vi "Clear Plots Without Assigned Variables.vi"(8 "error in":errorcluster, 10 "Plot Channel Configurations":T3[](array[typedef]), 11 "Plot Data In":T1[](array[typedef])) -> (0 "error out":errorcluster, 3 "Plot Data Out":T1[](array[typedef]))   [LabVIEW 2017, in "DTacq Plot Display Library.lvlib"]
doc: "Clear out old data, which can result from changing the number of plots."
uses:
  DTacq Plot Display Library.lvlib
  Plot Data--Cluster.ctl
  Network Shared Variables/Typedefs/X and Y Variant Arrays--Cluster.ctl
  Typedefs/Plot Channel Configruation--Cluster.ctl
  Network Shared Variables/Shared Variables Library.lvlib
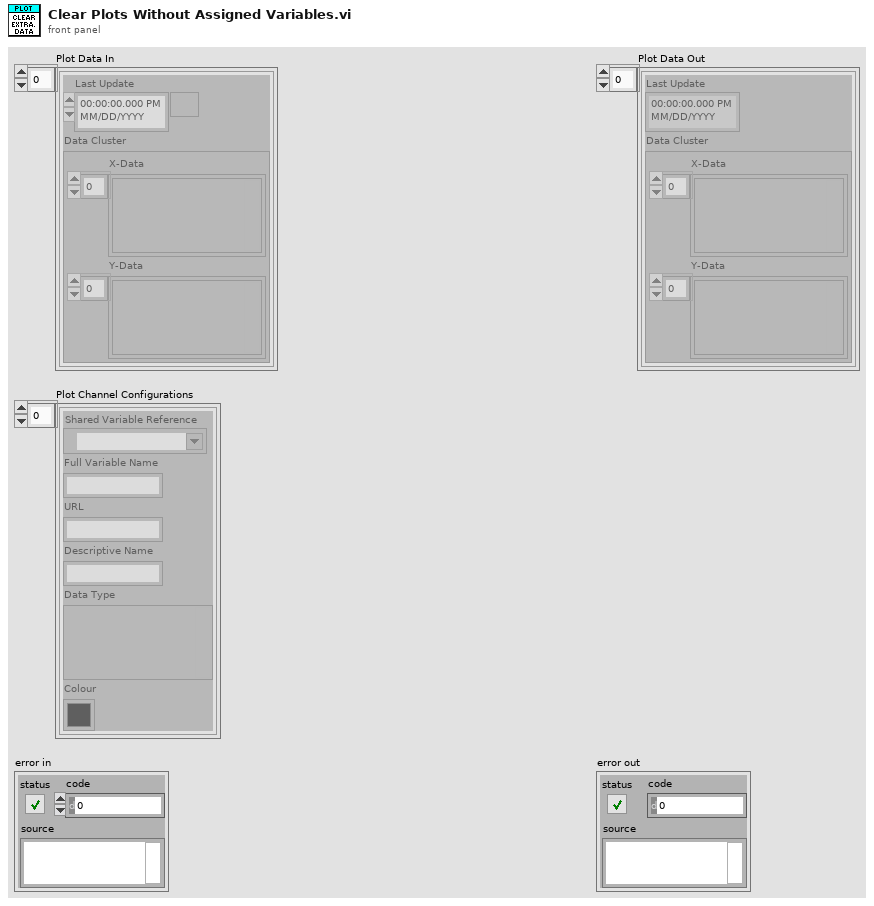
[diagram p1: front panel]
types:
  T1 = typedef "DTacq Plot Display Library.lvlib/Plot Data--Cluster.ctl" = cluster{"Last Update":timestamp, "Data Cluster":T2}
  T2 = typedef "Shared Variables Library.lvlib/X and Y Variant Arrays--Cluster.ctl" = cluster{"X-Data":variant[], "Y-Data":variant[]}
  T3 = typedef "DTacq Plot Display Library.lvlib/Plot Channel Configruation--Cluster.ctl" = cluster{"Shared Variable Reference":refnum<k21>, "Full Variable Name":string, "URL":string, "Descriptive Name":string, "Data Type":variant, "Colour":u32}
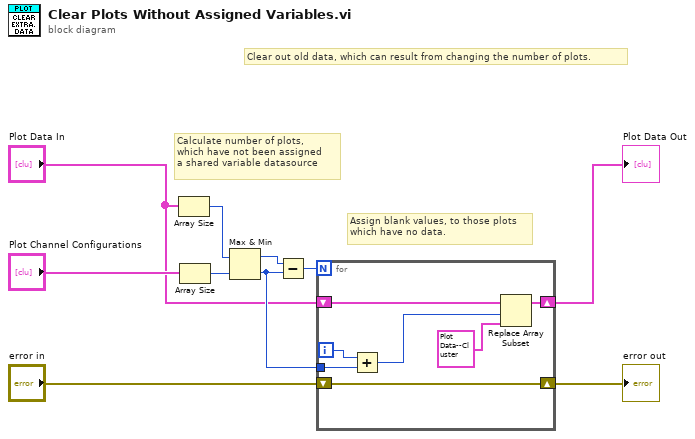
[diagram p0: block diagram]
diagram:
  # "Clear out old data, which can result from changing the number of plots."
  # "Assign blank values, to those plots\nwhich have no data."
  # "Calculate number of plots,\nwhich have not been assigned \na shared variable datasource"
  n1 = Array Size(array="Plot Data In") -> (size(s)=w5:i32)
  n2 = Array Size(array="Plot Channel Configurations") -> (size(s)=w4:i32)
  n3 = Max & Min(x=w5, y=w4) -> (max(x,y)=w8:i32, min(x,y)=w10:i32)
  n4 = Subtract(x=w8, y=w10) -> (x-y=w9:i32)
  n5 = for {
    N: w9 -> [_]
    shift-right: [w17] -> w7
    shift-left: "error in" -> [w17]
    tunnel: w10 -> [w15]
    shift-right: [w11] -> w1
    shift-left: "Plot Data In" -> [w14]
    i -> [w16]
    n6 = Add(x=w16, y=w15) -> (x+y=w13:i32)
    n7 = Replace Array Subset(array=w14, new element=T1 {"Last Update"=timestamp(0 s since 1904-01-01), "Data Cluster"={"X-Data"=[], "Y-Data"=[]}}, index=w13) -> (w11:T1[])
  }
  "error out" <- w7
  "Plot Data Out" <- w1
